vi "MPU_Stick_Serial_Port_Emulator.vi"(8 "error in (no error)":errorcluster, 11 "MPU_Stick_Globals":T1) -> ()   [LabVIEW 2017]
uses:
  Controls/MPU_Stick_Globals.ctl
  Controls/IMU_Configuration_References.ctl
  Controls/MP_Comp_Filter_Constants_References.ctl
  Controls/MD_Threshold_References.ctl
  Controls/MD_Type_References.ctl
  Controls/LED_Configuration_References.ctl
  Controls/Primary_References.ctl
  Controls/MPU_Stick_Queues.ctl
  Controls/MPU_Stick_Queue_Element.ctl
  Controls/MPU_Stick_Queue_Commands.ctl
  Classes/ADCP.lvclass
  <vilib>/Utility/file.llb/Read Delimited Spreadsheet (string).vi
  MPU_Stick_Read_Serial_Port_Emulator.vi
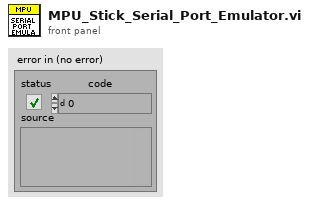
[diagram p1: front panel]
types:
  T1 = typedef "MPU_Stick_Globals.ctl" = cluster{"IMU_configuration_references":T2, "MP_Comp_Filter_Constants_References":T3, "MD_Threshold_References":T4, "MD_Type_References":T5, "LED_Configuration_References":T6, "Primary_references":T7, "MPU_Stick_Queues":T8, "ADCP":refnum<vi>}
  T2 = typedef "IMU_Configuration_References.ctl" = cluster{"Get all IMU configurations":refnum<vi>, "Set all IMU configurations":refnum<vi>, "Get sampling frequency":refnum<vi>, "Set sampling frequency":refnum<vi>, "Get calibration point count":refnum<vi>, "Set calibration point count":refnum<vi>, "Get calibration interval":refnum<vi>, "Set calibration interval":refnum<vi>, "Get Gyroscope bandwidth":refnum<vi>, "Set Gyroscope bandwidth":refnum<vi>, "Get Gyroscope F.S. Value":refnum<vi>, "Set Gyroscope F.S. Value":refnum<vi>, "Get Accelerometer bandwidth":refnum<vi>, "Set Accelerometer bandwidth":refnum<vi>, "Get Accelerometer F.S. Value":refnum<vi>, "Set Accelerometer F.S. Value":refnum<vi>, "Sampling frequency (Hz)":refnum<vi>, "Calibration point count":refnum<vi>, "Calibration interval (ms)":refnum<vi>, "IMU Gyroscope bandwidth":refnum<vi>, "IMU Gyroscope F.S. value":refnum<vi>, "IMU Accelerometer bandwidth":refnum<vi>, "IMU Accelerometer F.S. value":refnum<vi>}
  T3 = typedef "MP_Comp_Filter_Constants_References.ctl" = cluster{"Set pitch filter constant":refnum<vi>, "Get pitch filter constant":refnum<vi>, "Set roll filter constant":refnum<vi>, "Get roll filter constant":refnum<vi>, "Pitch filter constant":refnum<vi>, "Roll filter constant":refnum<vi>}
  T4 = typedef "MD_Threshold_References.ctl" = cluster{"Yaw threshold (U)":refnum<vi>, "Yaw threshold (L)":refnum<vi>, "Pitch threshold (U)":refnum<vi>, "Pitch. threshold (L)":refnum<vi>, "Roll threshold (U)":refnum<vi>, "Roll threshold (L)":refnum<vi>, "Z gyro. threshold (U)":refnum<vi>, "Z gyro. threshold (L)":refnum<vi>, "Y gyro. threshold (U)":refnum<vi>, "Y gyro. threshold (L)":refnum<vi>, "X gyro. threshold (U)":refnum<vi>, "X gyro. threshold (L)":refnum<vi>, "Z accel. threshold (U)":refnum<vi>, "Z accel. threshold (L)":refnum<vi>, "Y accel. threshold (U)":refnum<vi>, "Y accel. threshold (L)":refnum<vi>, "X accel. threshold (U)":refnum<vi>, "X accel. threshold (L)":refnum<vi>, "Set all Motion detection threshold configurations":refnum<vi>, "Get yaw threshold (upper)":refnum<vi>, "Get yaw threshold (lower)":refnum<vi>, "Get pitch threshold (upper)":refnum<vi>, "Get pitch threshold (lower)":refnum<vi>, "Get roll threshold (upper)":refnum<vi>, "Get roll threshold (lower)":refnum<vi>, "Get Z gyro threshold (upper)":refnum<vi>, "Get Z gyro threshold (lower)":refnum<vi>, "Get Y gyro threshold (upper)":refnum<vi>, "Get Y gyro threshold (lower)":refnum<vi>, "Get X gyro threshold (upper)":refnum<vi>, "Get X gyro threshold (lower)":refnum<vi>, "Get Z accel threshold (upper)":refnum<vi>, "Get Z accel threshold (lower)":refnum<vi>, "Get Y accel threshold (upper)":refnum<vi>, "Get Y accel threshold (lower)":refnum<vi>, "Get X accel threshold (upper)":refnum<vi>, "Get X accel threshold (lower)":refnum<vi>, "Get all Motion detection threshold configurations":refnum<vi>, "Set yaw threshold (upper)":refnum<vi>, "Set yaw threshold (lower)":refnum<vi>, "Set pitch threshold (upper)":refnum<vi>, "Set pitch threshold (lower)":refnum<vi>, "Set roll threshold (upper)":refnum<vi>, "Set roll threshold (lower)":refnum<vi>, "Set Z gyro threshold (upper)":refnum<vi>, "Set Z gyro threshold (lower)":refnum<vi>, "Set Y gyro threshold (upper)":refnum<vi>, "Set Y gyro threshold (lower)":refnum<vi>, "Set X gyro threshold (upper)":refnum<vi>, "Set X gyro threshold (lower)":refnum<vi>, "Set Z accel threshold (upper)":refnum<vi>, "Set Z accel threshold (lower)":refnum<vi>, "Set Y accel threshold (upper)":refnum<vi>, "Set Y accel threshold (lower)":refnum<vi>, "Set X accel threshold (upper)":refnum<vi>, "Set X accel threshold (lower)":refnum<vi>}
  T5 = typedef "MD_Type_References.ctl" = cluster{"Yaw threshold type":refnum<vi>, "Pitch threshold type":refnum<vi>, "Roll threshold type":refnum<vi>, "Z gyro threshold type":refnum<vi>, "Y gyro threshold type":refnum<vi>, "X gyro threshold type":refnum<vi>, "Z accel threshold type":refnum<vi>, "Y accel threshold type":refnum<vi>, "X accel threshold type":refnum<vi>, "Set all Motion detection type configurations":refnum<vi>, "Get all Motion detection type configurations":refnum<vi>, "Set yaw threshold type":refnum<vi>, "Get yaw threshold type":refnum<vi>, "Set pitch threshold type":refnum<vi>, "Get pitch threshold type":refnum<vi>, "Set roll threshold type":refnum<vi>, "Get roll threshold type":refnum<vi>, "Set Z gyroscope threshold type":refnum<vi>, "Get Z gyroscope threshold type":refnum<vi>, "Set Y gyroscope threshold type":refnum<vi>, "Get Y gyroscope threshold type":refnum<vi>, "Set X gyroscope threshold type":refnum<vi>, "Get X gyroscope threshold type":refnum<vi>, "Set Z accel threshold type":refnum<vi>, "Get Z accel threshold type":refnum<vi>, "Set Y accel threshold type":refnum<vi>, "Get Y accel threshold type":refnum<vi>, "Get X accel threshold type":refnum<vi>, "Set X accel threshold type":refnum<vi>}
  T6 = typedef "LED_Configuration_References.ctl" = cluster{"Get all LED configurations":refnum<vi>, "Set all LED configurations":refnum<vi>, "Get LED3 configuration":refnum<vi>, "Set LED3 configuration":refnum<vi>, "Get LED2 configuration":refnum<vi>, "Set LED2 configuration":refnum<vi>, "Get LED1 configuration":refnum<vi>, "Set LED1 configuration":refnum<vi>, "LED3 Configuration":refnum<vi>, "LED2 Configuration":refnum<vi>, "LED1 Configuration":refnum<vi>}
  T7 = typedef "Primary_References.ctl" = cluster{"3D View Image":refnum<vi>, "Plot":refnum<vi>, "Graph / 3D view tab control":refnum<vi>, "MP Reset":refnum<vi>, "Calibrate IMU":refnum<vi>, "Plot Parameter List":refnum<vi>, "Remove Parameter from Plot":refnum<vi>, "Add Parameter to Plot":refnum<vi>, "Parameter to monitor":refnum<vi>, "Yaw motion detection output":refnum<vi>, "Pitch motion detection output":refnum<vi>, "Roll motion detection output":refnum<vi>, "Z gyro motion detection output":refnum<vi>, "Y gyro motion detection output":refnum<vi>, "X gyro motion detection output":refnum<vi>, "Z accel motion detection output":refnum<vi>, "Y accel motion detection output":refnum<vi>, "X accel motion detection output":refnum<vi>, "Yaw angle (filter) (degrees)":refnum<vi>, "Pitch angle (filter) (degrees)":refnum<vi>, "Roll angle (filter) (degrees)":refnum<vi>, "Yaw angle (gyro) (degrees)":refnum<vi>, "Pitch angle (gyro) (degrees)":refnum<vi>, "Roll angle (gyro) (degrees)":refnum<vi>, "Yaw angle (accel) (degrees)":refnum<vi>, "Pitch angle (accel) (degrees)":refnum<vi>, "Roll angle (accel) (degrees)":refnum<vi>, "Z gyroscope reading (DPS)":refnum<vi>, "Y gyroscope reading (DPS)":refnum<vi>, "X gyroscope reading (DPS)":refnum<vi>, "Z accelerometer reading (G)":refnum<vi>, "Y accelerometer reading (G)":refnum<vi>, "X accelerometer reading (G)":refnum<vi>, "Save all config.":refnum<vi>, "Write all config.":refnum<vi>, "Read all config.":refnum<vi>, "Tab Control":refnum<vi>, "Baud Rate":refnum<vi>, "COM Port":refnum<vi>, "Time (ms)":refnum<vi>, "Value (Units)":refnum<vi>, "Exit Application":refnum<vi>, "Connect Device":refnum<vi>, "Progress Bar":refnum<vi>, "Get Range & Offset":refnum<vi>, "Range":refnum<vi>, "Offset":refnum<vi>, "Set Range & Offset":refnum<vi>, "Parameter name":refnum<vi>, "Plot time (ms)":refnum<vi>, "Plot value":refnum<vi>}
  T8 = typedef "MPU_Stick_Queues.ctl" = cluster{"UI Event Handler":refnum<queue>, "3D View Updater":refnum<queue>, "Plot Updater":refnum<queue>, "Serial Port Reader":refnum<queue>, "UI Indicators Updater":refnum<queue>}
  T9 = cluster{"Parameter Names":string[], "Parameter Values":string[], "Time (ms)":dbl}
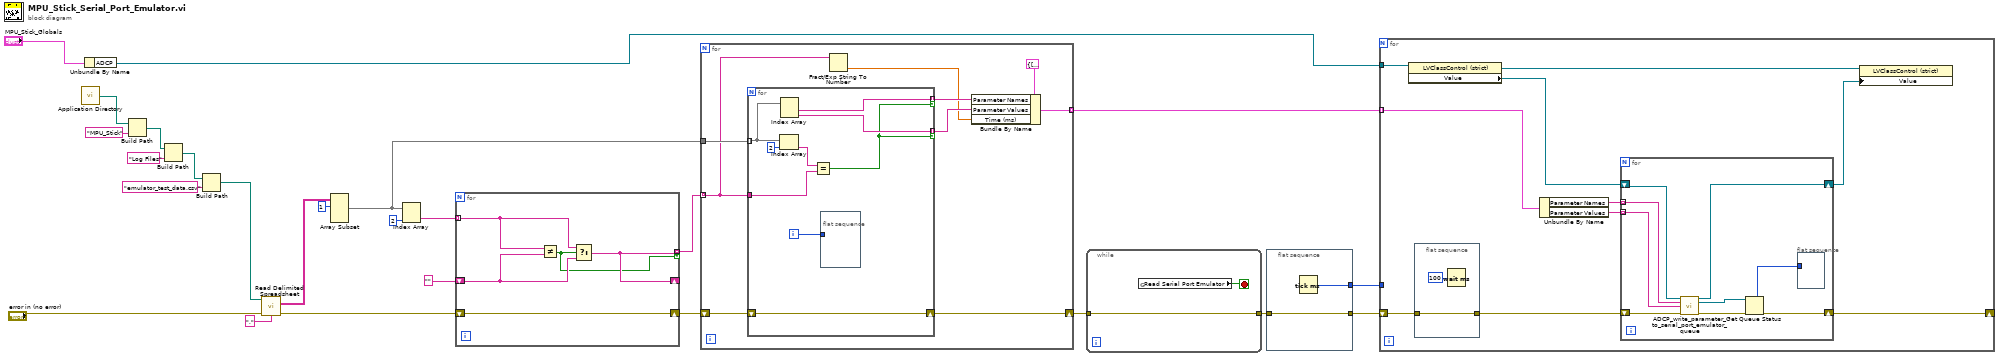
[diagram p0: block diagram]
diagram:
  n1 = call <vilib>:"Application Directory.vi"() -> ("Application Directory"=w25:path)
  n2 = Unbundle By Name("MPU_Stick_Globals") -> ("ADCP"=w1:refnum<vi>)
  n3 = Build Path(base path=w25, name or relative path="MPU_Stick") -> (appended path=w23:path)
  n4 = Build Path(base path=w23, name or relative path="Log Files") -> (appended path=w21:path)
  n5 = Build Path(base path=w21, name or relative path="emulator_test_data.csv") -> (appended path=w18:path)
  n6 = call-poly <vilib>:"Read Delimited Spreadsheet.vi"("file path (dialog if empty)"=w18, "error in (no error)"="error in (no error)", "delimiter (\\t)"="," ("delimiter (\\t)")) -> ("all rows"=w16:string[][], "error out"=w11:errorcluster)  [unwired: 7 in, 4 out]
  n7 = Array Subset(array=w16, index (row)=1 ("index")) -> (w5:string[][])  [unwired: 3 in]
  n8 = Index Array(array=w5, index (col)=2 ("disabled index (col)")) -> (element=w10:string[])  [unwired: 1 in]
  n9 = for {
    tunnel: w10 -> [w29] mode=indexing
    shift-right: [w27] -> _
    shift-left: "" -> [w28]
    shift-right: [w30] -> w8
    shift-left: w11 -> [w30]
    tunnel: [w27] -> w6 mode=indexing if=w26
    n10 = Not Equal?(x=w29, y=w28) -> (x != y?=w26:bool)
    n11 = Select(t=w29, s=w26, f=w28) -> (s? t:f=w27:string)
  }
  n12 = for {
    shift-right: [w38] -> w7
    shift-left: w8 -> [w39]
    tunnel: w6 -> [w33] mode=indexing
    tunnel: w5 -> [w37]
    tunnel: [w31] -> w2 mode=indexing
    n13 = for {
      shift-right: [w48] -> w38
      shift-left: w39 -> [w48]
      tunnel: w37 -> [w44] mode=indexing
      tunnel: w33 -> [w45]
      tunnel: [w43] -> w35 mode=indexing if=w41
      tunnel: [w42] -> w34 mode=indexing if=w41
      i -> [w40]
      n14 = Index Array(array=w44, index=2) -> (element=w46:string)
      n15 = Index Array(array=w44) -> (element #1=w43:string, element #2=w42:string)  [unwired: 2 in]
      n16 = Equal?(x=w46, y=w45) -> (x = y?=w41:bool)
      n17 = flat-sequence {
        tunnel: w40 -> [_]
        frame #0 {
        }
      }
    }
    n18 = Fract/Exp String To Number(string=w33) -> (number=w32:dbl)  [unwired: 3 in, 1 out]
    n19 = Bundle By Name(cluster=T9 {"Parameter Names"=[], "Parameter Values"=[], "Time (ms)"=0.0}, "Parameter Names"=w35, "Parameter Values"=w34, "Time (ms)"=w32) -> (w31:T9)
  }
  n20 = while {
    tunnel: w7 -> [w50]
    tunnel: [w50] -> w13
    stop <- w49 stop-if-true
    n21 = global read "MPU_Stick_Read_Serial_Port_Emulator.vi" "Read Serial Port Emulator"() -> (w49:bool)
  }
  n22 = flat-sequence {
    tunnel: w13 -> [w52]
    tunnel: [w52] -> w4
    tunnel: [w51] -> w3
    frame #0 {
      n23 = Tick Count (ms)() -> (millisecond timer value=w51:u32)
    }
  }
  n24 = for {
    shift-right: [w53] -> _
    shift-left: w4 -> [w62]
    tunnel: w3 -> [_]
    tunnel: w2 -> [w60] mode=indexing
    tunnel: w1 -> [w57]
    n25 = property class="LVClassControl (strict)"(reference=w57) -> (reference out=w55:refnum<vi>, "Value"=w56:refnum<class "ADCP.lvclass">)  [unwired: 1 in, 1 out]
    n26 = flat-sequence {
      tunnel: w62 -> [w64]
      tunnel: [w64] -> w61
      frame #0 {
        n27 = Wait (ms)(milliseconds to wait=u32 100) -> ()  [unwired: 1 out]
      }
    }
    n28 = Unbundle By Name(w60) -> ("Parameter Names"=w59:string[], "Parameter Values"=w58:string[])
    n29 = for {
      tunnel: w59 -> [w71] mode=indexing
      tunnel: w58 -> [w70] mode=indexing
      shift-right: [w69] -> w54
      shift-left: w56 -> [w72]
      shift-right: [w67] -> w53
      shift-left: w61 -> [w73]
      n30 = call "ADCP_write_parameter_to_serial_port_emulator_queue.vi"("ADCP In"=w72, "Parameter Name"=w71, "Parameter Value"=w70, "error in (no error)"=w73) -> ("ADCP out"=w69:refnum<class "ADCP.lvclass">, "Queue Out"=w66:refnum<queue>, "error out"=w68:errorcluster)  [unwired: 9 in]
      n31 = Get Queue Status(queue=w66, error in (no error)=w68) -> (error out=w67:errorcluster, # elements in queue=w65:i32)  [unwired: 1 in, 6 out]
      n32 = flat-sequence {
        tunnel: w65 -> [_]
        frame #0 {
        }
      }
    }
    n33 = property class="LVClassControl (strict)"(reference=w55, "Value"=w54) -> ()  [unwired: 1 in, 2 out]
  }
